vi "GVSView Pic Set TF Data.vi"(7 "sAction":string, 8 "pVIRef":refnum<vi>, 9 "sData":string) -> ()   [LabVIEW 2013]
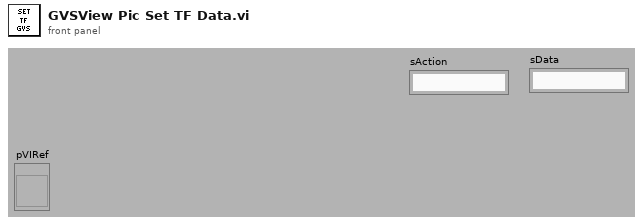
[diagram p1: front panel]
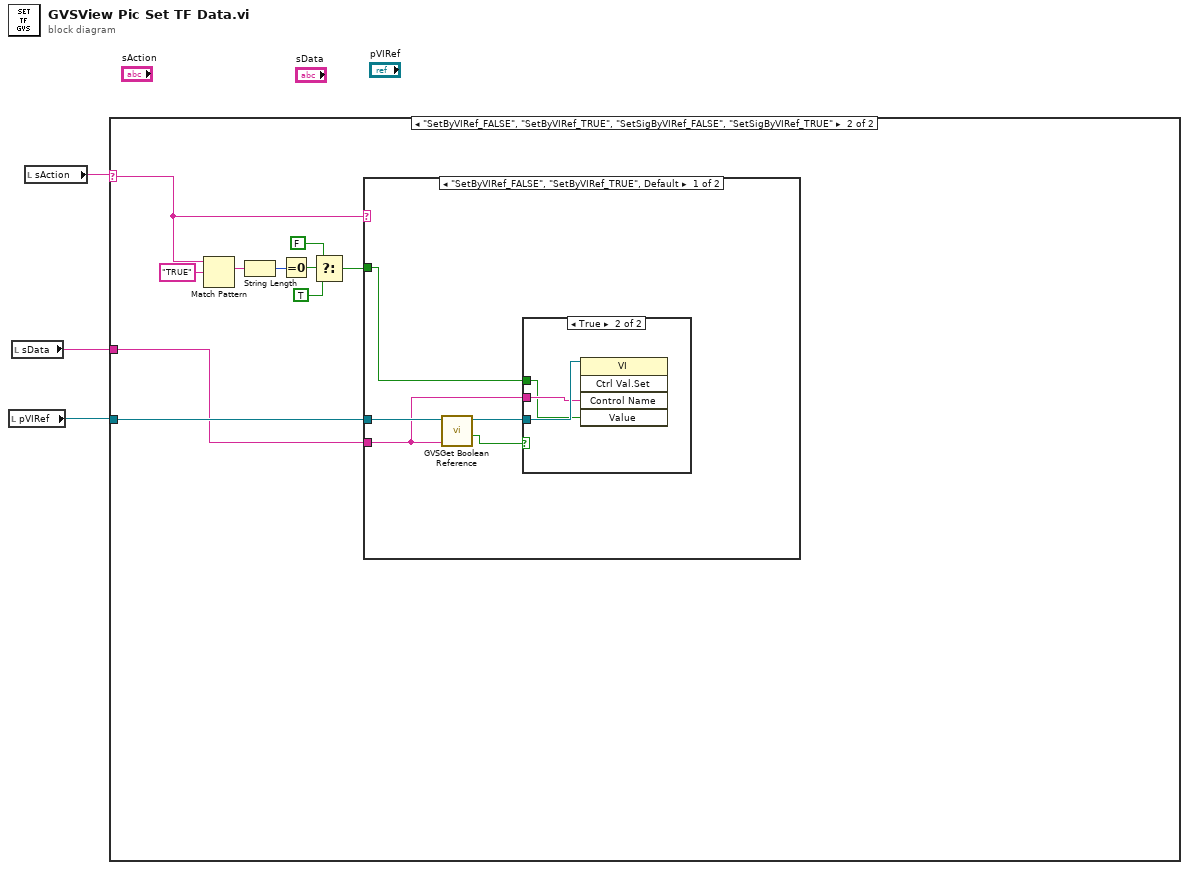
[diagram p0: block diagram]
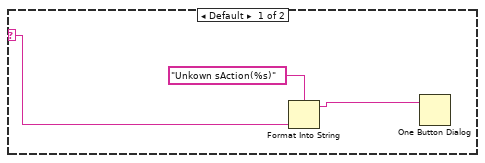
[diagram p2: hidden frame]
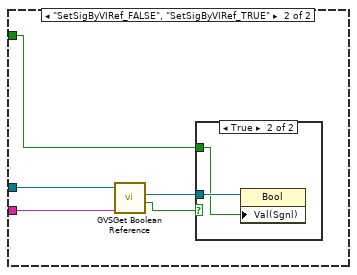
[diagram p4: hidden frame]
diagram:
  n1 = local read "pVIRef"() -> (w1:refnum<vi>)
  n2 = local read "sData"() -> (w2:string)
  n3 = local read "sAction"() -> (w3:string)
  n4 = case shown="\"SetByVIRef_FALSE\", \"SetByVIRef_TRUE\", \"SetSigByVIRef_FALSE\", \"SetSigByVIRef_TRUE\"" w3 {
    selector: w3 -> [w5 w7]
    tunnel: w2 -> [_ w15]
    tunnel: w1 -> [_ w16]
    frame Default {
      n5 = Format Into String(format string="Unkown sAction(%s)", w5) -> (resulting string=w4:string)  [unwired: 2 in, 1 out]
      n6 = One Button Dialog(message=w4) -> ()  [unwired: 1 in, 1 out]
    }
    frame "SetByVIRef_FALSE", "SetByVIRef_TRUE", "SetSigByVIRef_FALSE", "SetSigByVIRef_TRUE" {
      n7 = Match Pattern(string=w7, regular expression="TRUE") -> (match substring=w13:string)  [unwired: 1 in, 3 out]
      n8 = String Length(string=w13) -> (length=w12:i32)
      n9 = Equal To 0?(x=w12) -> (x = 0?=w11:bool)
      n10 = Select(t=FALSE, s=w11, f=TRUE) -> (s? t:f=w8:bool)
      n11 = case shown="\"SetByVIRef_FALSE\", \"SetByVIRef_TRUE\", Default" w7 {
        tunnel: w16 -> [w20 w28]
        tunnel: w15 -> [w17 w27]
        tunnel: w8 -> [w19 w25]
        frame "SetByVIRef_FALSE", "SetByVIRef_TRUE", Default {
          n12 = call "GVSGet Boolean Reference.vi"("Label Name"=w17, "VI Refnum"=w20) -> ("Boolean"=w21:bool, "VI Refnum Out"=w18:refnum<vi>)  [unwired: 7 in, 1 out]
          n13 = case shown="True" w21 {
            tunnel: w19 -> [_ w22]
            tunnel: w18 -> [_ w24]
            tunnel: w17 -> [_ w23]
            frame False {
            }
            frame True {
              n14 = invoke class="VI" method="Ctrl Val.Set"(reference=w24, "Control Name"=w23, "Value"=w22) -> ()  [unwired: 2 in, 5 out]
            }
          }
        }
        frame "SetSigByVIRef_FALSE", "SetSigByVIRef_TRUE" {
          n15 = call "GVSGet Boolean Reference.vi"("Label Name"=w27, "VI Refnum"=w28) -> ("Boolean"=w26:bool, "Boolean Ref"=w29:refnum<vi>)  [unwired: 7 in, 1 out]
          n16 = case shown="True" w26 {
            tunnel: w29 -> [_ w31]
            tunnel: w25 -> [_ w30]
            frame False {
            }
            frame True {
              n17 = property class="Bool"(reference=w31, "Val(Sgnl)"=w30) -> ()  [unwired: 1 in, 2 out]
            }
          }
        }
      }
    }
  }
